vi "R1Master.vi"(6 "LabVIEW Web Service":refnum<class "Web Service.lvclass">=refnum) -> ()   [LabVIEW 2016]
uses:
  <vilib>/wsapi/Web Service.lvclass
  <vilib>/Platform/TimedLoop/XDataNode/XDataNode.xnode
  <vilib>/Platform/TimedLoop/XDataNode/nitl_modes.ctl
  <vilib>/Platform/TimedLoop/XDataNode/XDNodeRunTimeDep.lvlib
  <vilib>/Platform/TimedLoop/XDataNode/wakeup.ctl
  <vilib>/Platform/TimedLoop/XDataNode/timing_clust.ctl
  <vilib>/Platform/TimedLoop/XDataNode/loadnilvce.vi
  Controls/pH_Manual Standard.ctl
  Controls/ISE_CF.ctl
  Controls/Tri State Control.ctl
  Controls/R1SBR_SetParams.ctl
  Controls/pH_SetParams Standard.ctl
panel:
  out "NH4 Probe Reading, mgN/L":dbl
  out "error out (pH)":errorcluster
  in  "R1ORPSlope":dbl=1000.0
  in  "R1ORPIntercept":dbl
  in  "R1pHSlope":dbl=1066.018
  in  "R1pHIntercept":dbl=-6.03166
  out "AcidPumpTotalizer":dbl
  out "BasePumpTotalizer":dbl
  in  "R1 pH_Switch":bool=TRUE
  in  "R1pH_SetParams":T1={"Set Point"=7.5, "Tolerance"=0.1, "Pump Time On, secs"=4.0}
  in  "R1pH_Manual":cluster{"Acid Pump":bool, "Base Pump":bool}
  out "pH":cluster{"Signal":dbl, "Value":dbl}
  in  "R1_K_SetParams":T3={"Equil Approach Set point, mV/min"=0.5, "Equil Approach dt, s"=30.0, "Interference Correction Factors"=[], "Detect Equilibrium?"=TRUE, "Probe Intercept"=-7.6147, "Probe Slope"=0.01624, "Baseline"=154.0, "Detection Limit, M"=2e-06}
  in  "R1_NH4_SetParams":T3={"Equil Approach Set point, mV/min"=1.0, "Equil Approach dt, s"=30.0, "Interference Correction Factors"=[{"Correction Factor"=0.002, "Ion"="Na", "Correct For Ion?"=FALSE}, {"Correction Factor"=0.1, "Ion"="K", "Correct For Ion?"=FALSE}], "Detect Equilibrium?"=FALSE, "Probe Intercept"=-3.418, "Probe Slope"=0.01672, "Baseline"=-85.37, "Detection Limit, M"=2e-06}
  in  "R1_Na_SetParams":T3={"Equil Approach Set point, mV/min"=0.5, "Equil Approach dt, s"=30.0, "Interference Correction Factors"=[{"Correction Factor"=1.6, "Ion"="K", "Correct For Ion?"=TRUE}], "Detect Equilibrium?"=TRUE, "Probe Intercept"=-6.9115, "Probe Slope"=0.03178, "Baseline"=90.1097, "Detection Limit, M"=2e-06}
  out "R1NaISE":T5 {"Steady State?" items=["False", "True", "NaN", ""]}
  out "R1NH4ISE":T5 {"Steady State?" items=["False", "True", "NaN", ""]}
  out "R1 K ISE":T5 {"Steady State?" items=["False", "True", "NaN", ""]}
  in  "R1SBR_SetParams":T6=[{"Phase"="Plug Feed", "Time, min"=0.0, "SBR_Manual"={"Media Pump"=TRUE, "Water Pump"=TRUE, "Effluent Pump"=FALSE, "Release Valve"=FALSE, "Gas Pump"=FALSE}}, {"Phase"="Mixed Feed", "Time, min"=100.0, "SBR_Manual"={"Media Pump"=TRUE, "Water Pump"=TRUE, "Effluent Pump"=FALSE, "Release Valve"=FALSE, "Gas Pump"=TRUE}}, {"Phase"="Mixed W/O Feed", "Time, min"=0.0, "SBR_Manual"={"Media Pump"=FALSE, "Water Pump"=FALSE, "Effluent Pump"=FALSE, "Release Valve"=FALSE, "Gas Pump"=TRUE}}, {"Phase"="Settle", "Time, min"=3.0, "SBR_Manual"={"Media Pump"=FALSE, "Water Pump"=FALSE, "Effluent Pump"=FALSE, "Release Valve"=FALSE, "Gas Pump"=FALSE}}, {"Phase"="Decant", "Time, min"=4.0, "SBR_Manual"={"Media Pump"=FALSE, "Water Pump"=FALSE, "Effluent Pump"=TRUE, "Release Valve"=TRUE, "Gas Pump"=FALSE}}, {"Phase"="Idle", "Time, min"=1.0, "SBR_Manual"={"Media Pump"=FALSE, "Water Pump"=FALSE, "Effluent Pump"=FALSE, "Release Valve"=FALSE, "Gas Pump"=FALSE}}] {"Time, min" min=1.0}
  in  "R1SBRManual":T7
  in  "R1 SBR_Switch":bool=TRUE
  out "error out (Master)":errorcluster
  out "error out (Data)":errorcluster
  out "error out (SBR)":errorcluster
  out "Graph":T8(graph)
  out "Timestamp":string
  out "Status":string="Off"
  out "Cycle Time Elapsed":dbl
  out "Phase Time Elapsed":dbl
  # "Don't press the run button!"
  # "Use the web service input terminal to call the VIs on the Service subpalette of the Web Services palette. Do not remove it from the connector pane unless you don't need access to the palette."
  # "Any additional terminals added to the connector pane of a startup VI will be ignored."
  # "Don't press the run button!"
  # "pH Control"
  # "SBR Control"
  # "If On, Automate SBR Cycle"
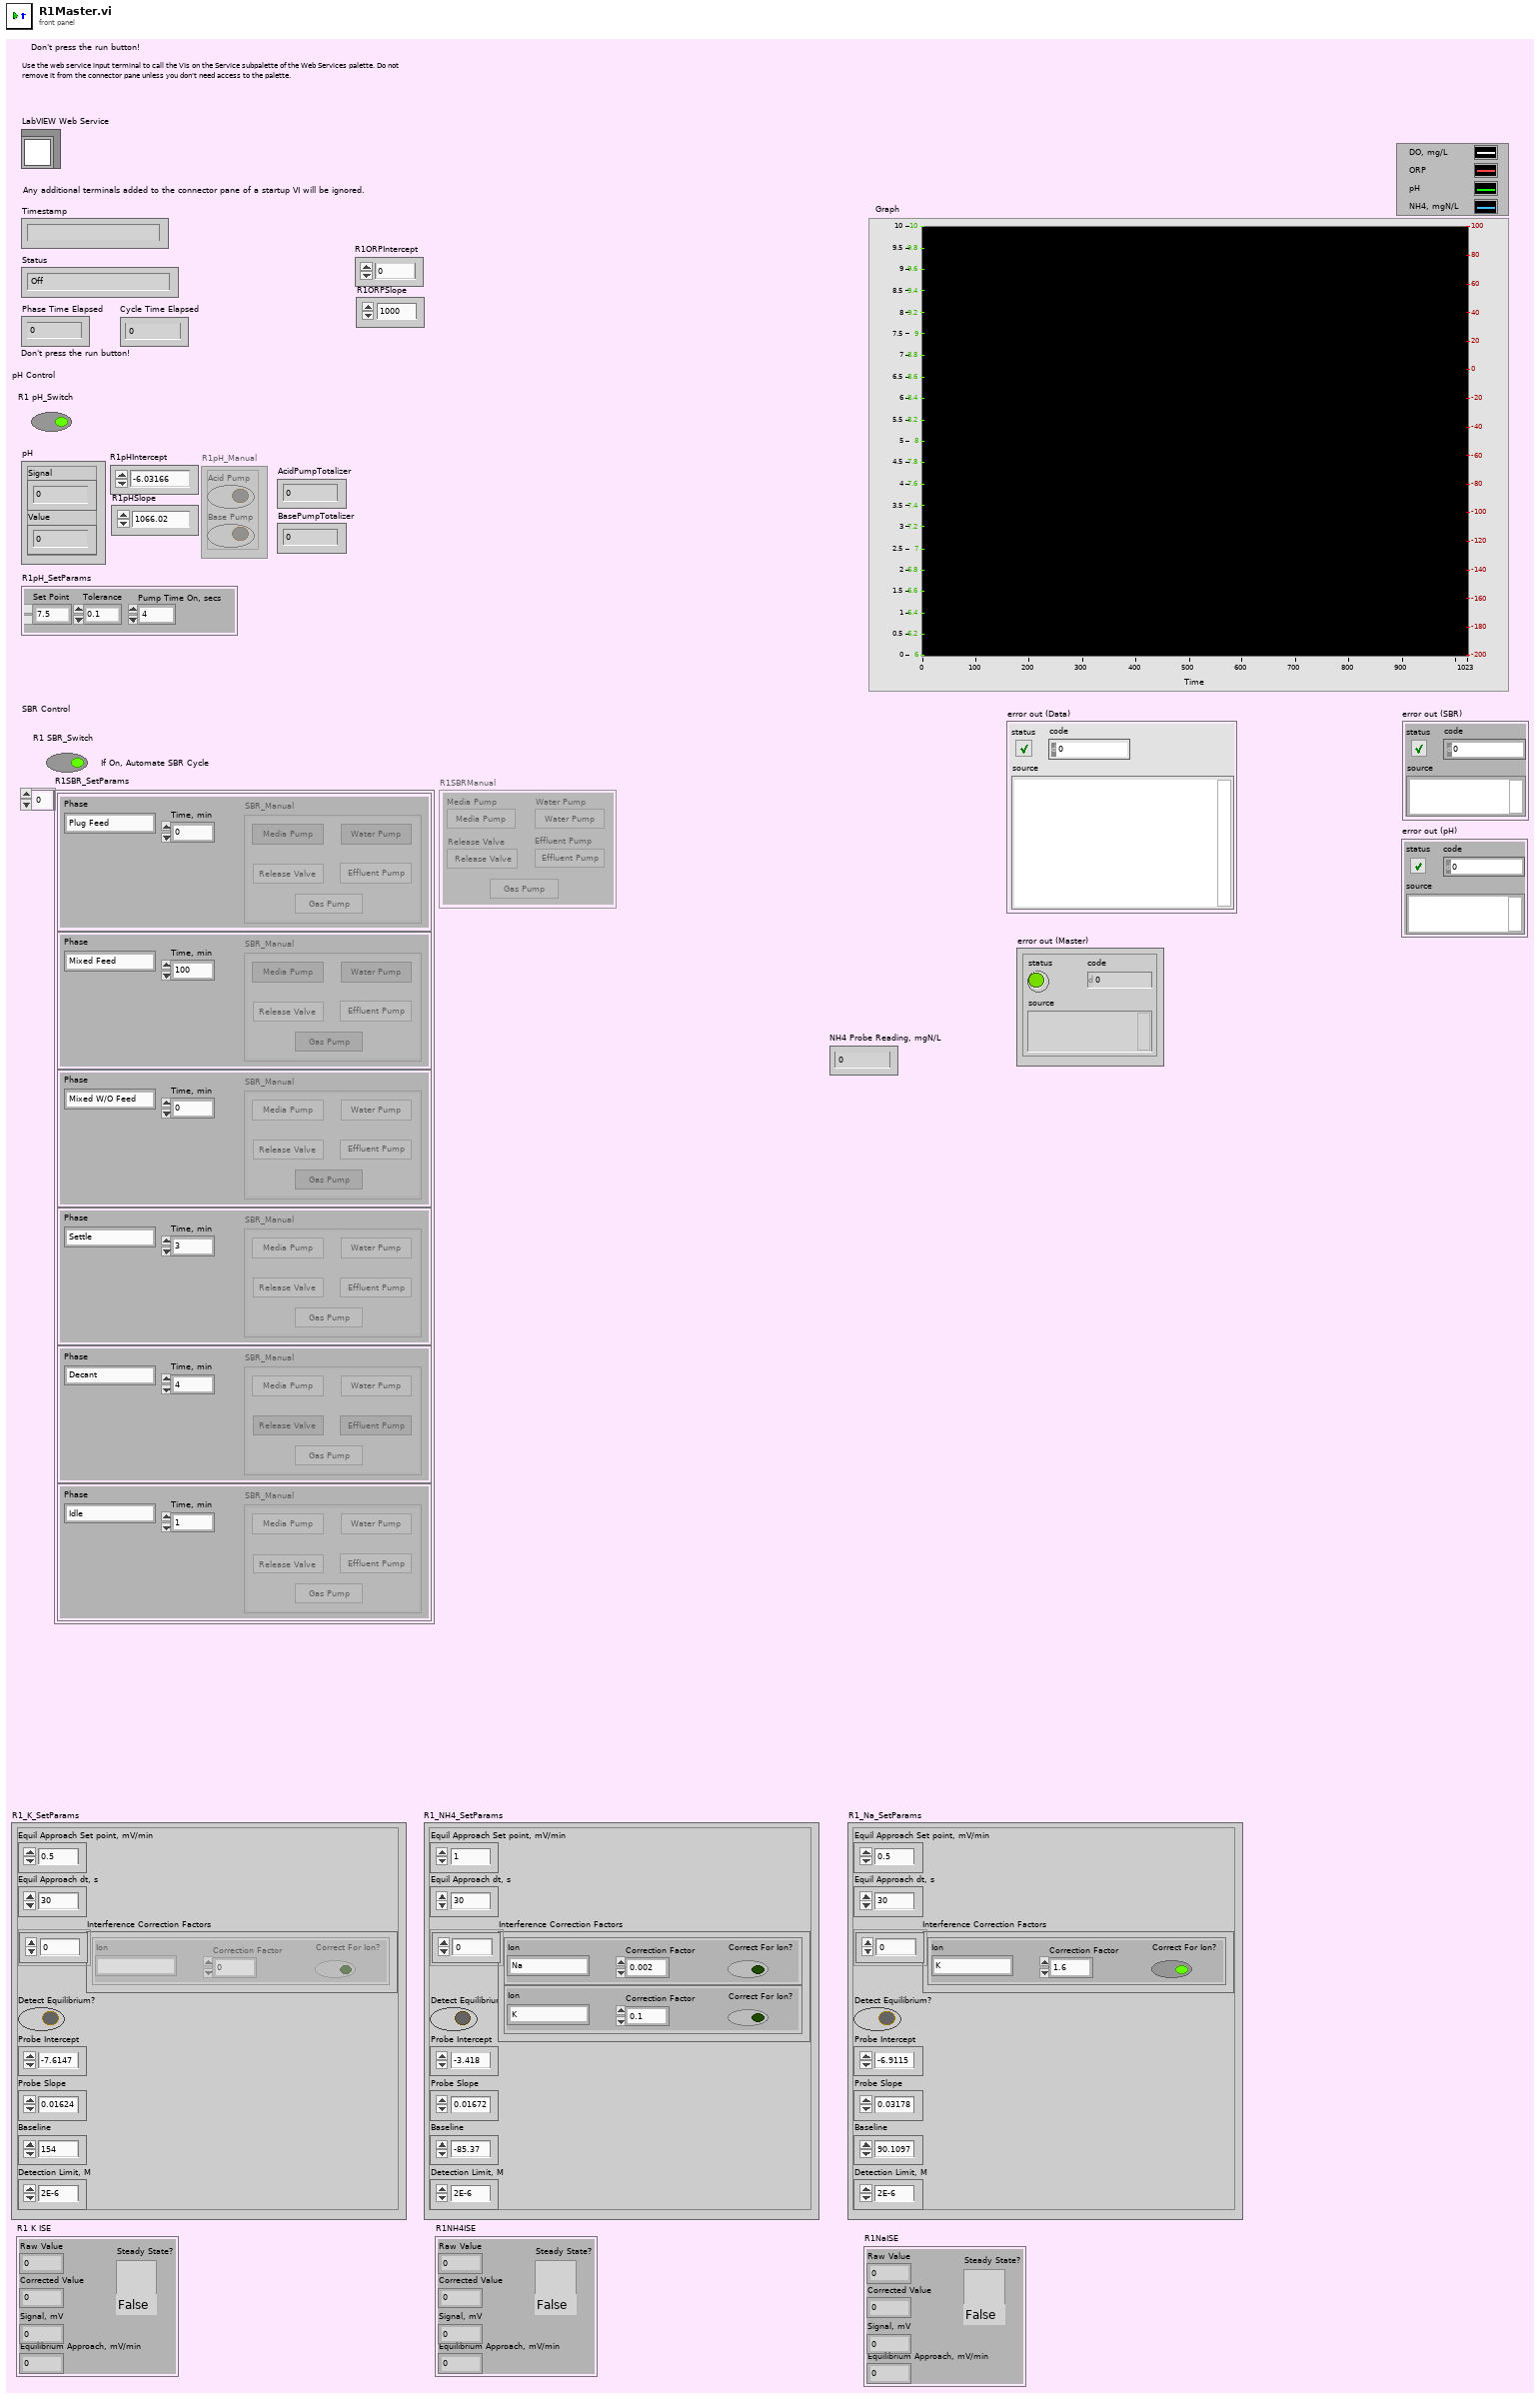
[diagram p1: front panel]
types:
  T1 = typedef "pH_SetParams Standard.ctl" = cluster{"Set Point":dbl, "Tolerance":dbl, "Pump Time On, secs":dbl}
  T2 = typedef "ISE_CF.ctl" = cluster{"Correction Factor":dbl, "Ion":string, "Correct For Ion?":bool}
  T3 = cluster{"Equil Approach Set point, mV/min":dbl, "Equil Approach dt, s":dbl, "Interference Correction Factors":T2[], "Detect Equilibrium?":bool, "Probe Intercept":dbl, "Probe Slope":dbl, "Baseline":dbl, "Detection Limit, M":dbl}
  T4 = typedef "Tri State Control.ctl" = u16
  T5 = cluster{"Raw Value":dbl, "Corrected Value":dbl, "Signal, mV":dbl, "Equilibrium Approach, mV/min":dbl, "Steady State?":T4}
  T6 = typedef "R1SBR_SetParams.ctl" = cluster{"Phase":string, "Time, min":dbl, "SBR_Manual":cluster{"Media Pump":bool, "Water Pump":bool, "Effluent Pump":bool, "Release Valve":bool, "Gas Pump":bool}}[]
  T7 = cluster{"Media Pump":bool, "Water Pump":bool, "Effluent Pump":bool, "Release Valve":bool, "Gas Pump":bool}
  T8 = cluster{"Value":dbl, "Value, UNITS HERE":dbl, "Value":dbl, "Corrected Value":dbl}
  T9 = typedef "XDNodeRunTimeDep.lvlib/timing_clust.ctl" = cluster{"Expected End [f-1]":u64, "Actual End [f-1]":u64, "Finished Late? [f-1]":bool, "Expected End [i-1]":u64, "Actual End [i-1]":u64, "Finished Late? [i-1]":bool, "Expected Start [i]":u64, "Actual Start [i]":u64, "Expected Start [f]":u64, "Actual Start [f]":u64, "Source Name":string, "Structure Name":string, "Period":i64, "Deadline":i64, "Offset":i64, "Start":i64, "Priority":i32, "Timeout":i32, "Mode":T10, "Wakeup Reason":T11, "Error":errorcluster, "Source Type":string, "Secondary Source Type":string, "Global End Time":u64, "Global Start Time":u64, "Frame Duration":u64, "Iteration Duration":u64, "Assigned CPU":i32, "I/O Scan Engine Mode":u32}
  T10 = typedef "XDNodeRunTimeDep.lvlib/nitl_modes.ctl" = enum32{"No Change", "Process missed periods, maintain original phase", "Discard missed periods, maintain original phase", "Process missed periods, ignore original phase", "Discard missed periods, ignore original phase"}
  T11 = typedef "XDNodeRunTimeDep.lvlib/wakeup.ctl" = enum32{"Normal", "Aborted", "Asynchronous wakeup", "Timing source error", "Timed loop error", "Timeout"}
  T12 = enum8{"Enabled", "Disabled", "Disabled and Grayed Out"}
  T13 = typedef "pH_Manual Standard.ctl" = cluster{"Acid Pump":bool, "Base Pump":bool}
  T14 = cluster{"Set Point, mg/L":dbl, "Tolerance, mg/L":dbl, "N2 Valve Gain":dbl, "Air Valve Gain":dbl}
  T15 = cluster{"Set Point, mgN/L":dbl, "Tolerance, mgN/L":dbl, "Pump Gain":dbl, "Max Volume/Cycle, mL":dbl}
  T16 = cluster{"Signal, mA":dbl, "Value, UNITS HERE":dbl}
  T17 = cluster{"Value":dbl, "Value, UNITS HERE":dbl, "Value":dbl, dbl}
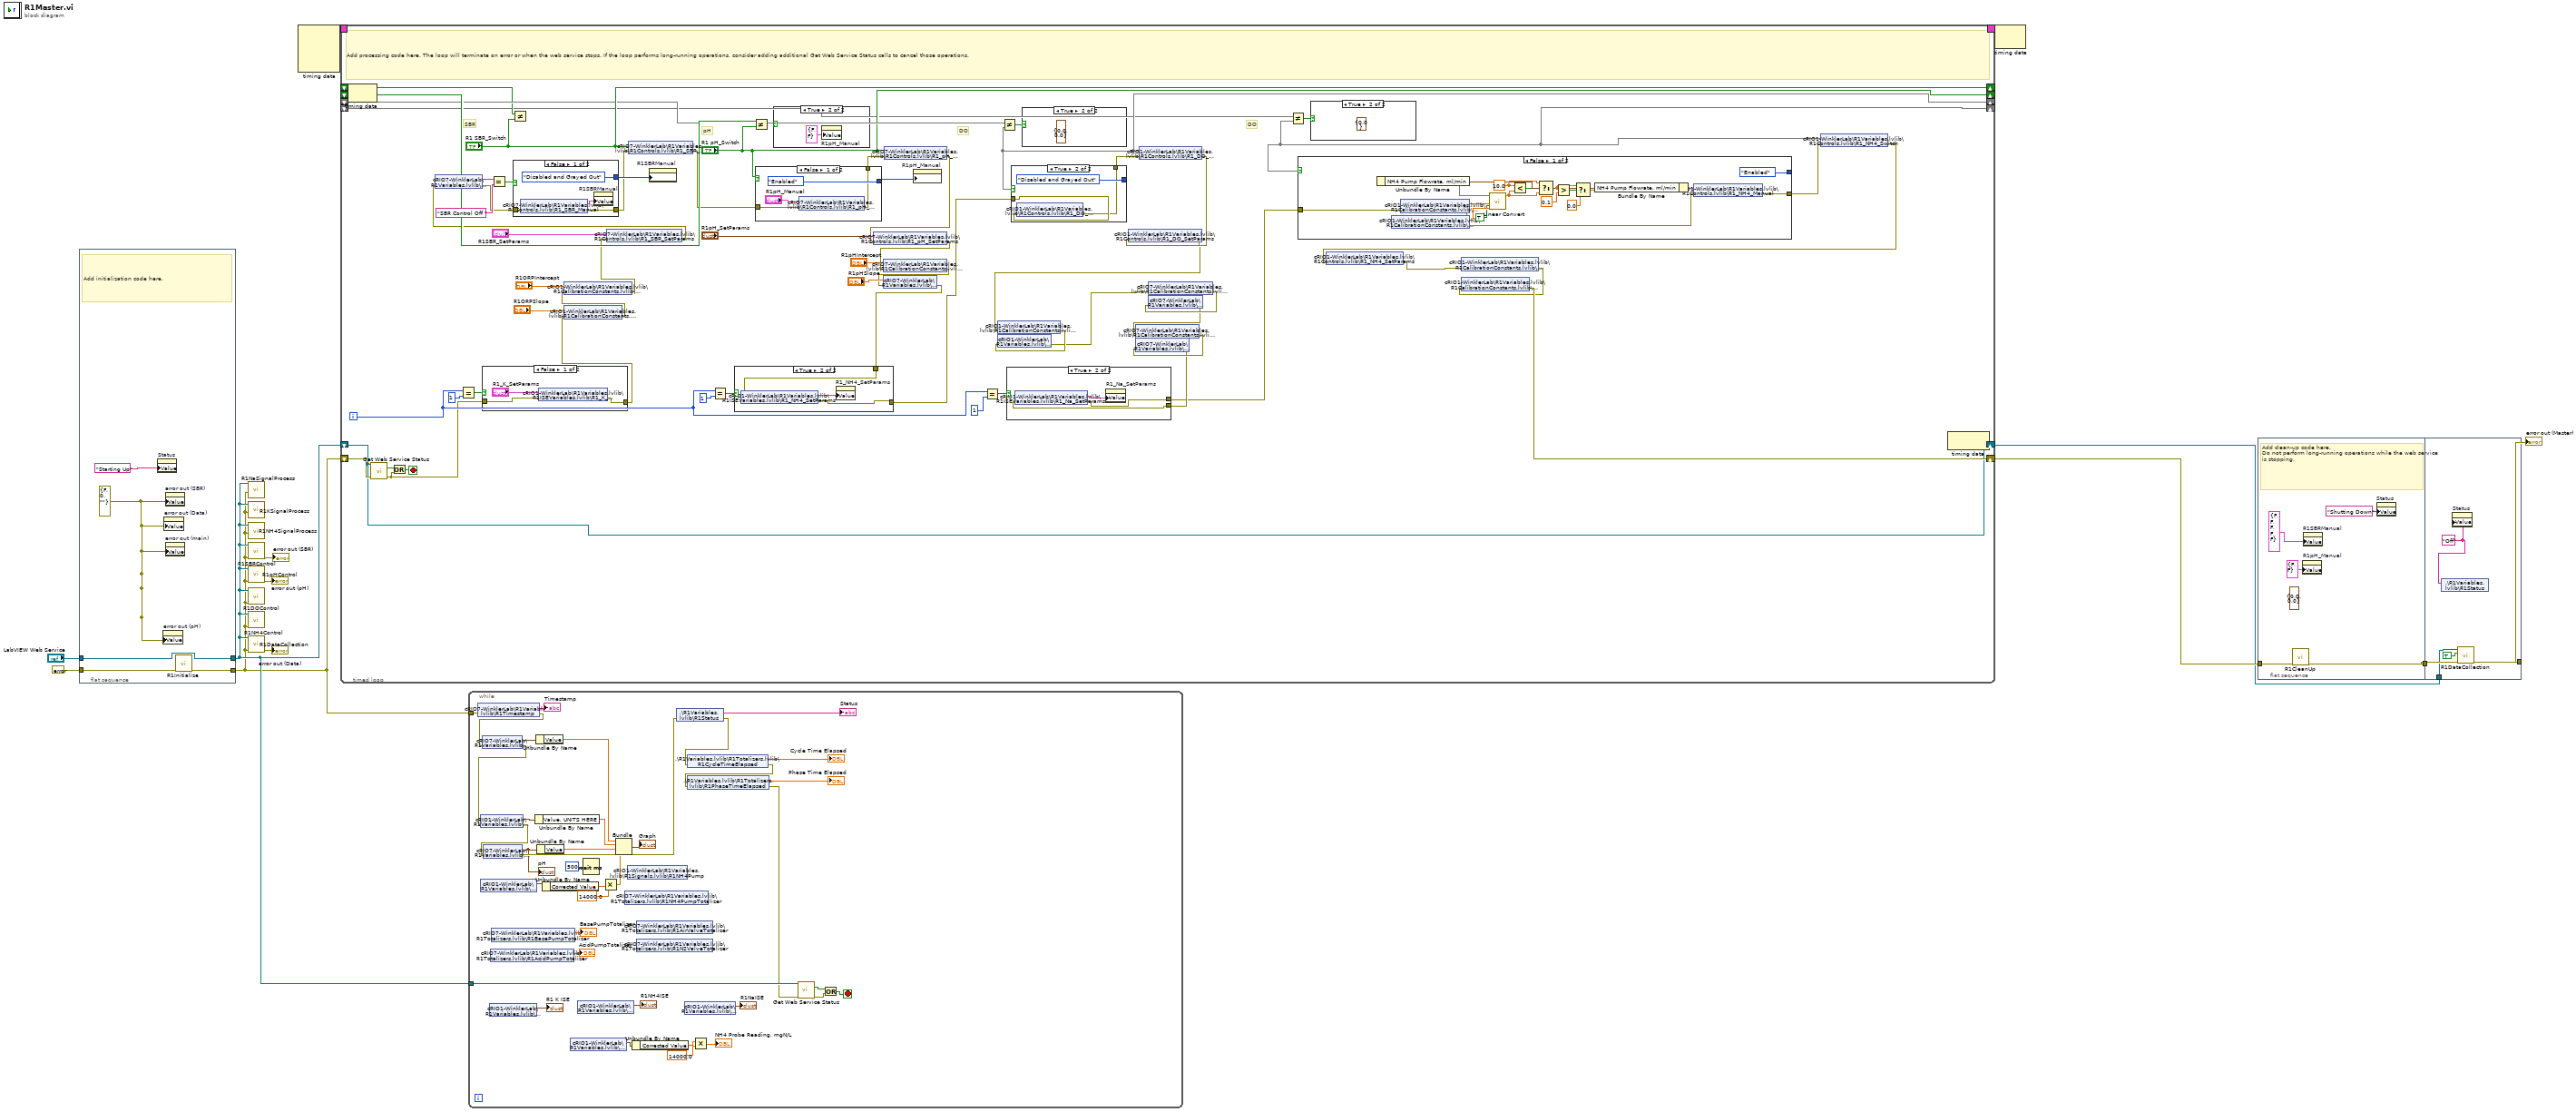
[diagram p0: block diagram]
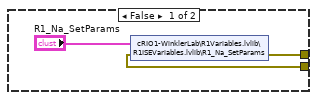
[diagram p2: hidden frame]
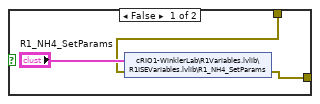
[diagram p3: hidden frame]
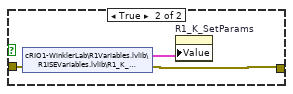
[diagram p4: hidden frame]
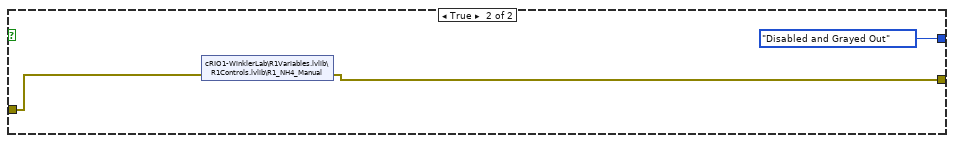
[diagram p6: hidden frame]
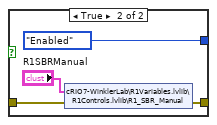
[diagram p9: hidden frame]
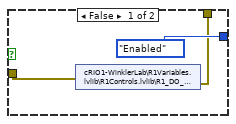
[diagram p10: hidden frame]
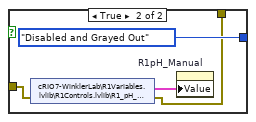
[diagram p11: hidden frame]
diagram:
  n1 = flat-sequence {
    tunnel: "LabVIEW Web Service" -> [w16]
    tunnel: errorcluster {"status"=FALSE, "code"=0, "source"=""} ("error constant") -> [w18]
    tunnel: [w17] -> w2
    tunnel: [w16] -> w3
    frame #0 {
      w14 = errorcluster {"status"=FALSE, "code"=0, "source"=""} ("error out (SBR)")
      # "Add initialization code here."
      n2 = property on="Status" class="Str"("Value"="Starting Up" ("Status")) -> ()  [unwired: 2 in, 2 out]
      n3 = property on="error out (pH)" class="Clust (strict)"("Value"=w14) -> ()  [unwired: 2 in, 2 out]
      n4 = property on="error out (Data)" class="Clust (strict)"("Value"=w14) -> ()  [unwired: 2 in, 2 out]
      n5 = property on="error out (SBR)" class="Clust (strict)"("Value"=w14) -> ()  [unwired: 2 in, 2 out]
      n6 = property on="error out (main)" class="Clust (strict)"("Value"=w14) -> ()  [unwired: 2 in, 2 out]
      n7 = call "R1Initialize.vi"("error in (no error)"=w18) -> ("error out"=w17:errorcluster)  [unwired: 10 in]
    }
  }
  n8 = call "R1NaSignalProcess.vi"("error"=w2, "LabVIEW Web Service"=w3) -> ()  [unwired: 9 in, 1 out]
  n9 = call "R1KSignalProcess.vi"("error"=w2, "LabVIEW Web Service"=w3) -> ()  [unwired: 9 in, 1 out]
  n10 = call "R1NH4SignalProcess.vi"("error"=w2, "LabVIEW Web Service"=w3) -> ()  [unwired: 9 in, 1 out]
  n11 = call "R1SBRControl.vi"("error constant"=w2, "LabVIEW Web Service"=w3) -> ("error out"=→"error out (SBR)":errorcluster)  [unwired: 9 in]
  n12 = call "R1pHControl.vi"("error constant"=w2, "LabVIEW Web Service"=w3) -> ("error out"=→"error out (pH)":errorcluster)  [unwired: 9 in]
  n13 = call "R1DOControl.vi"("error constant"=w2, "LabVIEW Web Service"=w3) -> ()  [unwired: 9 in, 1 out]
  n14 = call "R1NH4Control.vi"("error constant"=w2, "LabVIEW Web Service"=w3) -> ()  [unwired: 9 in, 1 out]
  n15 = call "R1DataCollection.vi"("error constant"=w2, "LabVIEW Web Service"=w3) -> ("error out"=→"error out (Data)":errorcluster)  [unwired: 9 in]
  n16 = node-c288() -> (w10:T9)  [unwired: 4 in]
  n17 = timed-loop {
    shift-right: [w80] -> w11
    shift-left: w2 -> [w83]
    shift-right: [w79] -> w1
    shift-left: w3 -> [w79]
    timing: w10 -> [_]
    timing-out: [_] -> w9
    shift-right: ["R1 SBR_Switch"] -> _
    shift-left: _ -> [w86]
    shift-right: ["R1 pH_Switch"] -> _
    shift-left: _ -> [w90]
    shift-right: _ -> [w88]
    shift-left: _ -> [w89]
    shift-right: _ -> [w78]
    shift-left: _ -> [w77]
    i -> [w85]
    stop <- w82 stop-if-true
    # "DO"
    # "DO"
    # "pH"
    # "SBR"
    # "Add processing code here. The loop will terminate on error or when the web service stops. If the loop performs long-running operations, consider adding additional Get Web Service Status calls to cancel those operations."
    n18 = node-c288() -> ()  [unwired: 1 in, 1 out]
    n19 = call <vilib>:"Get Web Service Status.vi"("LabVIEW Web Service"=w79, "error in (no error)"=w83) -> ("service stopping?"=w84:bool, "error out"=w81:errorcluster)  [unwired: 11 in, 1 out]
    n20 = Or(x=w84, y=w81) -> (x .or. y?=w82:bool)
    n21 = Equal?(x=w85, y=1) -> (x = y?=w63:bool)
    n22 = case shown="False" w63 {
      tunnel: w81 -> [w105 w108]
      tunnel: [w104 w107] -> w45
      frame False {
        n23 = shared-variable "cRIO1-WinklerLab\\R1Variables.lvlib\\R1ISEVariables.lvlib\\R1_K_SetParams"("R1_K_SetParams", error in=w105) -> (error out=w104:errorcluster)
      }
      frame True {
        n24 = shared-variable "cRIO1-WinklerLab\\R1Variables.lvlib\\R1ISEVariables.lvlib\\R1_K_SetParams"(error in=w108) -> (w109:T3, error out=w107:errorcluster)
        n25 = property on="R1_K_SetParams" class="Clust (strict)"("Value"=w109) -> ()  [unwired: 2 in, 2 out]
      }
    }
    n26 = Not Equal?(x=w86, y="R1 SBR_Switch") -> ()  [unwired: 1 out]
    n27 = shared-variable "cRIO1-WinklerLab\\R1Variables.lvlib\\R1CalibrationConstants.lvlib\\R1ORPSlope"("R1ORPSlope", error in=w45) -> (error out=w44:errorcluster)
    n28 = shared-variable "cRIO1-WinklerLab\\R1Variables.lvlib\\R1CalibrationConstants.lvlib\\R1ORPIntercept"("R1ORPIntercept", error in=w44) -> (error out=w43:errorcluster)
    n29 = shared-variable "cRIO7-WinklerLab\\R1Variables.lvlib\\R1Controls.lvlib\\R1_SBR_SetParams"("R1SBR_SetParams", error in=w43) -> (error out=w42:errorcluster)
    n30 = shared-variable "cRIO7-WinklerLab\\R1Variables.lvlib\\R1Status"(error in=w42) -> (w67:string, error out=w41:errorcluster)
    n31 = Equal?(x=w67, y="SBR Control Off " ("string")) -> (x = y?=w65:bool)
    n32 = case shown="False" w65 {
      tunnel: [T12."Disabled and Grayed Out" ("Disabled") T12."Enabled" ("Disabled")] -> w72
      tunnel: w41 -> [w137 w141]
      tunnel: [w136 w140] -> w40
      frame False {
        n33 = shared-variable "cRIO7-WinklerLab\\R1Variables.lvlib\\R1Controls.lvlib\\R1_SBR_Manual"(error in=w137) -> (w138:T7, error out=w136:errorcluster)
        n34 = property on="R1SBRManual" class="Clust (strict)"("Value"=w138) -> ()  [unwired: 2 in, 2 out]
      }
      frame True {
        n35 = shared-variable "cRIO7-WinklerLab\\R1Variables.lvlib\\R1Controls.lvlib\\R1_SBR_Manual"("R1SBRManual", error in=w141) -> (error out=w140:errorcluster)
      }
    }
    n36 = shared-variable "cRIO7-WinklerLab\\R1Variables.lvlib\\R1Controls.lvlib\\R1_SBR_Switch"("R1 SBR_Switch", error in=w40) -> (error out=w39:errorcluster)
    n37 = property on="R1SBRManual" class="Clust (strict)"("DisabledEnum"=w72) -> ()  [unwired: 2 in, 2 out]
    n38 = Equal?(x=w85, y=1) -> (x = y?=w61:bool)
    n39 = Not Equal?(x=w90, y="R1 pH_Switch") -> (x != y?=w71:bool)
    n40 = case shown="False" "R1 pH_Switch" {
      tunnel: [T12."Enabled" ("Disabled") T12."Disabled and Grayed Out" ("Disabled")] -> w76
      tunnel: w39 -> [w152 w156]
      tunnel: [w151 w155] -> w38
      frame False {
        n41 = shared-variable "cRIO7-WinklerLab\\R1Variables.lvlib\\R1Controls.lvlib\\R1_pH_Manual"("R1pH_Manual", error in=w152) -> (error out=w151:errorcluster)
      }
      frame True {
        n42 = shared-variable "cRIO7-WinklerLab\\R1Variables.lvlib\\R1Controls.lvlib\\R1_pH_Manual"(error in=w156) -> (w157:T13, error out=w155:errorcluster)
        n43 = property on="R1pH_Manual" class="Clust (strict)"("Value"=w157) -> ()  [unwired: 2 in, 2 out]
      }
    }
    n44 = case shown="True" w71 {
      frame False {
      }
      frame True {
        n45 = property on="R1pH_Manual" class="Clust (strict)"("Value"=cluster{"Acid Pump":bool, "Base Pump":bool} {"Acid Pump"=FALSE, "Base Pump"=FALSE} ("R1pH_Manual")) -> ()  [unwired: 2 in, 2 out]
      }
    }
    n46 = shared-variable "cRIO7-WinklerLab\\R1Variables.lvlib\\R1Controls.lvlib\\R1_pH_Switch"("R1 pH_Switch", error in=w38) -> (error out=w37:errorcluster)
    n47 = shared-variable "cRIO7-WinklerLab\\R1Variables.lvlib\\R1Controls.lvlib\\R1_pH_SetParams"("R1pH_SetParams", error in=w37) -> (error out=w36:errorcluster)
    n48 = shared-variable "cRIO7-WinklerLab\\R1Variables.lvlib\\R1CalibrationConstants.lvlib\\R1pHIntercept"("R1pHIntercept", error in=w36) -> (error out=w35:errorcluster)
    n49 = shared-variable "cRIO7-WinklerLab\\R1Variables.lvlib\\R1CalibrationConstants.lvlib\\R1pHSlope"("R1pHSlope", error in=w35) -> (error out=w34:errorcluster)
    n50 = case shown="True" w61 {
      tunnel: w34 -> [w99 w102]
      tunnel: [w98 w101] -> w33
      frame False {
        n51 = shared-variable "cRIO1-WinklerLab\\R1Variables.lvlib\\R1ISEVariables.lvlib\\R1_NH4_SetParams"("R1_NH4_SetParams", error in=w99) -> (error out=w98:errorcluster)
      }
      frame True {
        n52 = shared-variable "cRIO1-WinklerLab\\R1Variables.lvlib\\R1ISEVariables.lvlib\\R1_NH4_SetParams"(error in=w102) -> (w103:T3, error out=w101:errorcluster)
        n53 = property on="R1_NH4_SetParams" class="Clust (strict)"("Value"=w103) -> ()  [unwired: 2 in, 2 out]
      }
    }
    n54 = property on="R1pH_Manual" class="Clust (strict)"("DisabledEnum"=w76) -> ()  [unwired: 2 in, 2 out]
    n55 = Equal?(x=w85, y=1) -> (x = y?=w58:bool)
    n56 = Not Equal?(x=w89, y=w88) -> (x != y?=w70:bool)
    n57 = case shown="True" w88 {
      tunnel: [T12."Enabled" ("Disabled") T12."Disabled and Grayed Out" ("Disabled")] -> w74
      tunnel: w33 -> [w145 w149]
      tunnel: [w144 w148] -> w32
      frame False {
        n58 = shared-variable "cRIO1-WinklerLab\\R1Variables.lvlib\\R1Controls.lvlib\\R1_DO_Manual"(error in=w145) -> (w146:cluster{"Air MFC":dbl, "N2 MFC":dbl}, error out=w144:errorcluster)
      }
      frame True {
        n59 = shared-variable "cRIO1-WinklerLab\\R1Variables.lvlib\\R1Controls.lvlib\\R1_DO_Manual"(error in=w149) -> (error out=w148:errorcluster)  [unwired: 1 out]
      }
    }
    n60 = case shown="True" w70 {
      frame False {
      }
      frame True {
        w134 = cluster{"Air MFC":dbl, "N2 MFC":dbl} {"Air MFC"=0.0, "N2 MFC"=0.0} ("R1DOManual")
      }
    }
    n61 = shared-variable "cRIO1-WinklerLab\\R1Variables.lvlib\\R1Controls.lvlib\\R1_DO_Switch"(w88, error in=w32) -> (error out=w31:errorcluster)
    n62 = shared-variable "cRIO1-WinklerLab\\R1Variables.lvlib\\R1Controls.lvlib\\R1_DO_SetParams"(error in=w31) -> (w73:T14, error out=w19:errorcluster)
    n63 = shared-variable "cRIO1-WinklerLab\\R1Variables.lvlib\\R1CalibrationConstants.lvlib\\R1AirIntercept"(error in=w19) -> (w51:dbl, error out=w30:errorcluster)
    n64 = shared-variable "cRIO1-WinklerLab\\R1Variables.lvlib\\R1CalibrationConstants.lvlib\\R1AirSlope"(error in=w30) -> (error out=w29:errorcluster)  [unwired: 1 in]
    n65 = shared-variable "cRIO7-WinklerLab\\R1Variables.lvlib\\R1CalibrationConstants.lvlib\\R1DOIntercept"(error in=w29) -> (w55:dbl, error out=w28:errorcluster)
    n66 = shared-variable "cRIO7-WinklerLab\\R1Variables.lvlib\\R1CalibrationConstants.lvlib\\R1DOSlope"(error in=w28) -> (w54:dbl, error out=w27:errorcluster)
    n67 = shared-variable "cRIO7-WinklerLab\\R1Variables.lvlib\\R1CalibrationConstants.lvlib\\R1N2Intercept"(error in=w27) -> (w53:dbl, error out=w26:errorcluster)
    n68 = shared-variable "cRIO7-WinklerLab\\R1Variables.lvlib\\R1CalibrationConstants.lvlib\\R1N2Slope"(error in=w26) -> (w52:dbl, error out=w25:errorcluster)
    n69 = case shown="True" w58 {
      tunnel: w25 -> [w93 w96]
      tunnel: [w92 w95] -> w24
      frame False {
        n70 = shared-variable "cRIO1-WinklerLab\\R1Variables.lvlib\\R1ISEVariables.lvlib\\R1_Na_SetParams"("R1_Na_SetParams", error in=w93) -> (error out=w92:errorcluster)
      }
      frame True {
        n71 = shared-variable "cRIO1-WinklerLab\\R1Variables.lvlib\\R1ISEVariables.lvlib\\R1_Na_SetParams"(error in=w96) -> (w97:T3, error out=w95:errorcluster)
        n72 = property on="R1_Na_SetParams" class="Clust (strict)"("Value"=w97) -> ()  [unwired: 2 in, 2 out]
      }
    }
    n73 = Not Equal?(x=w77, y=w78) -> (x != y?=w69:bool)
    n74 = case shown="False" w78 {
      tunnel: [T12."Enabled" ("Disabled") T12."Disabled and Grayed Out" ("Disabled")] -> w68
      tunnel: w24 -> [w114 w131]
      tunnel: [w111 w130] -> w23
      frame False {
        w122 = 10.0
        n75 = Unbundle By Name() -> (w125:cluster{"NH4 Pump Flowrate, ml/min":dbl}, "NH4 Pump Flowrate, ml/min"=w123)
        n76 = shared-variable "cRIO1-WinklerLab\\R1Variables.lvlib\\R1CalibrationConstants.lvlib\\NH4PumpSlope"(error in=w114) -> (w128:dbl, error out=w113:errorcluster)
        n77 = shared-variable "cRIO1-WinklerLab\\R1Variables.lvlib\\R1CalibrationConstants.lvlib\\NH4PumpIntercept"(error in=w113) -> (w127:dbl, error out=w112:errorcluster)
        n78 = call "Linear Convert.vi"("Inverse?"=TRUE, "Intercept"=w127, "Slope"=w128, "Signal"=w123) -> ("Result"=w120:dbl)  [unwired: 7 in]
        n79 = Less?(x=w122, y=w120) -> (x < y?=w121:bool)
        n80 = Select(t=w122, s=w121, f=w120) -> (s? t:f=w118:dbl)
        n81 = Greater?(x=w118, y=0.1) -> (0:w119:bool)
        n82 = Select(t=w118, s=w119, f=0.0) -> (s? t:f=w116:dbl)
        n83 = Bundle By Name(cluster=w125, "NH4 Pump Flowrate, ml/min"=w116) -> (w124:cluster{})
        n84 = shared-variable "cRIO1-WinklerLab\\R1Variables.lvlib\\R1Controls.lvlib\\R1_NH4_Manual"(w124, error in=w112) -> (error out=w111:errorcluster)
      }
      frame True {
        n85 = shared-variable "cRIO1-WinklerLab\\R1Variables.lvlib\\R1Controls.lvlib\\R1_NH4_Manual"(error in=w131) -> (w132:cluster{"NH4 Pump Flowrate, ml/min":dbl}, error out=w130:errorcluster)
      }
    }
    n86 = case shown="True" w69 {
      frame False {
      }
      frame True {
        w110 = cluster{"NH4 Pump Flowrate, ml/min":dbl} {"NH4 Pump Flowrate, ml/min"=0.0} ("R1NH4Manual")
      }
    }
    n87 = shared-variable "cRIO1-WinklerLab\\R1Variables.lvlib\\R1Controls.lvlib\\R1_NH4_Switch"(w78, error in=w23) -> (error out=w22:errorcluster)
    n88 = shared-variable "cRIO1-WinklerLab\\R1Variables.lvlib\\R1Controls.lvlib\\R1_NH4_SetParams"(error in=w22) -> (w46:T15, error out=w21:errorcluster)
    n89 = shared-variable "cRIO1-WinklerLab\\R1Variables.lvlib\\R1CalibrationConstants.lvlib\\NH4PumpIntercept"(error in=w21) -> (w50:dbl, error out=w20:errorcluster)
    n90 = shared-variable "cRIO1-WinklerLab\\R1Variables.lvlib\\R1CalibrationConstants.lvlib\\NH4PumpSlope"(error in=w20) -> (w49:dbl, error out=w80:errorcluster)
    n91 = node-c288() -> ()  [unwired: 1 in, 1 out]
  }
  n92 = while {
    tunnel: w3 -> [w194]
    tunnel: w2 -> [w185]
    stop <- w191 stop-if-true
    n93 = shared-variable "cRIO7-WinklerLab\\R1Variables.lvlib\\R1Timestamp"(error in=w185) -> (→"Timestamp":string, error out=w184:errorcluster)
    n94 = shared-variable "cRIO1-WinklerLab\\R1Variables.lvlib\\R1ISEVariables.lvlib\\R1_NH4_ISE"() -> (w176:T5)  [unwired: 1 in, 1 out]
    n95 = shared-variable "cRIO7-WinklerLab\\R1Variables.lvlib\\R1Signals.lvlib\\R1DO"(error in=w184) -> (w161:cluster{"Signal":dbl, "Value":dbl}, error out=w183:errorcluster)
    n96 = shared-variable "cRIO1-WinklerLab\\R1Variables.lvlib\\R1Signals.lvlib\\R1ORP"(error in=w183) -> (w169:T16, error out=w182:errorcluster)
    n97 = shared-variable "cRIO7-WinklerLab\\R1Variables.lvlib\\R1Signals.lvlib\\R1pH"(error in=w182) -> (w172:cluster{"Signal":dbl, "Value":dbl}, error out=w181:errorcluster)
    "pH" <- w172
    n98 = shared-variable "cRIO1-WinklerLab\\R1Variables.lvlib\\R1ISEVariables.lvlib\\R1_K_ISE"() -> (→"R1 K ISE":T5)  [unwired: 1 in, 1 out]
    n99 = shared-variable "cRIO7-WinklerLab\\R1Variables.lvlib\\R1Totalizers.lvlib\\R1AcidPumpTotalizer"() -> (→"AcidPumpTotalizer":dbl)  [unwired: 1 in, 1 out]
    n100 = shared-variable "cRIO7-WinklerLab\\R1Variables.lvlib\\R1Totalizers.lvlib\\R1BasePumpTotalizer"() -> (→"BasePumpTotalizer":dbl)  [unwired: 1 in, 1 out]
    n101 = Unbundle By Name(w169) -> ("Value, UNITS HERE"=w177:dbl)
    n102 = Unbundle By Name(w161) -> ("Value"=w195:dbl)
    n103 = Unbundle By Name(w172) -> ("Value"=w196:dbl)
    n104 = Unbundle By Name(w176) -> ("Corrected Value"=w175:dbl)
    n105 = shared-variable "cRIO1-WinklerLab\\R1Variables.lvlib\\R1ISEVariables.lvlib\\R1_NH4_ISE"() -> (w162:T5)  [unwired: 1 in, 1 out]
    n106 = shared-variable "cRIO1-WinklerLab\\R1Variables.lvlib\\R1ISEVariables.lvlib\\R1_NH4_ISE"() -> (→"R1NH4ISE":T5)  [unwired: 1 in, 1 out]
    n107 = Wait (ms)(milliseconds to wait=u32 500) -> ()  [unwired: 1 out]
    n108 = Multiply(x=14000.0, y=w175) -> (x*y=w174:dbl)
    n109 = Bundle("Value"=w195, "Value, UNITS HERE"=w177, "Value"=w196, w174) -> (→"Graph":T17)  [unwired: 1 in]
    n110 = shared-variable "cRIO7-WinklerLab\\R1Variables.lvlib\\R1Totalizers.lvlib\\R1NH4PumpTotalizer"() -> ()  [unwired: 1 in, 2 out]
    n111 = shared-variable "cRIO1-WinklerLab\\R1Variables.lvlib\\R1Signals.lvlib\\R1NH4Pump"() -> ()  [unwired: 1 in, 2 out]
    n112 = Unbundle By Name(w162) -> ("Corrected Value"=w163:dbl)
    n113 = shared-variable "cRIO7-WinklerLab\\R1Variables.lvlib\\R1Totalizers.lvlib\\R1AirValveTotalizer"() -> ()  [unwired: 1 in, 2 out]
    n114 = shared-variable "cRIO7-WinklerLab\\R1Variables.lvlib\\R1Totalizers.lvlib\\R1N2ValveTotalizer"() -> ()  [unwired: 1 in, 2 out]
    n115 = shared-variable ".\\R1Variables.lvlib\\R1Status"(error in=w181) -> (→"Status":string, error out=w180:errorcluster)
    n116 = shared-variable "cRIO1-WinklerLab\\R1Variables.lvlib\\R1ISEVariables.lvlib\\R1_Na_ISE"() -> (→"R1NaISE":T5)  [unwired: 1 in, 1 out]
    n117 = shared-variable ".\\R1Variables.lvlib\\R1Totalizers.lvlib\\R1CycleTimeElapsed"(error in=w180) -> (→"Cycle Time Elapsed":dbl, error out=w179:errorcluster)
    n118 = shared-variable ".\\R1Variables.lvlib\\R1Totalizers.lvlib\\R1PhaseTimeElapsed"(error in=w179) -> (→"Phase Time Elapsed":dbl, error out=w178:errorcluster)
    n119 = Multiply(x=w163, y=14000.0 ("x")) -> (x*y=→"NH4 Probe Reading, mgN/L":dbl)
    n120 = call <vilib>:"Get Web Service Status.vi"("LabVIEW Web Service"=w194, "error in (no error)"=w178) -> ("service stopping?"=w193:bool, "error out"=w192:errorcluster)  [unwired: 11 in, 1 out]
    n121 = Or(x=w193, y=w192) -> (x .or. y?=w191:bool)
  }
  n122 = node-c288(w9) -> ()  [unwired: 1 out]
  n123 = flat-sequence {
    tunnel: w11 -> [w201]
    tunnel: [w200] -> w7
    tunnel: w7 -> [w208]
    tunnel: [w207] -> w6
    tunnel: w1 -> [w204]
    frame #0 {
      w202 = cluster{"Air MFC":dbl, "N2 MFC":dbl} {"Air MFC"=0.0, "N2 MFC"=0.0} ("R1DOManual")
      # "Add clean-up code here.\nDo not perform long-running operations while the web service is stopping."
      n124 = call "R1CleanUp.vi"("error in (no error)"=w201) -> ("error out"=w200:errorcluster)  [unwired: 10 in]
      n125 = property on="R1pH_Manual" class="Clust (strict)"("Value"=cluster{"Acid Pump":bool, "Base Pump":bool} {"Acid Pump"=FALSE, "Base Pump"=FALSE} ("R1pH_Manual")) -> ()  [unwired: 2 in, 2 out]
      n126 = property on="R1SBRManual" class="Clust (strict)"("Value"=T7 {"Media Pump"=FALSE, "Water Pump"=FALSE, "Effluent Pump"=FALSE, "Release Valve"=FALSE, "Gas Pump"=FALSE} ("R1SBRManual")) -> ()  [unwired: 2 in, 2 out]
      n127 = property on="Status" class="Str"("Value"="Shutting Down" ("Status")) -> ()  [unwired: 2 in, 2 out]
    }
    frame #1 {
      w206 = "Off" ("Status")
      n128 = shared-variable ".\\R1Variables.lvlib\\R1Status"(w206) -> ()  [unwired: 1 in, 1 out]
      n129 = property on="Status" class="Str"("Value"=w206) -> ()  [unwired: 2 in, 2 out]
      n130 = call "R1DataCollection.vi"("error constant"=w208, "Write Once"=TRUE, "LabVIEW Web Service"=w204) -> ("error out"=w207:errorcluster)  [unwired: 8 in]
    }
  }
  "error out (Master)" <- w6
